vi "subIncrementAndGetProjectItem.vi"(8 "error in (no error)":errorcluster, 11 "BuildManager in":refnum<class "BuildManager.lvclass">) -> (0 "error out":errorcluster, 1 "Valid":bool, 3 "BuildManager out":refnum<class "BuildManager.lvclass">)   [LabVIEW 2019, in "SolutionBuilder.lvlib" / "BuildManager.lvclass"]
uses:
  BuildManager.lvclass
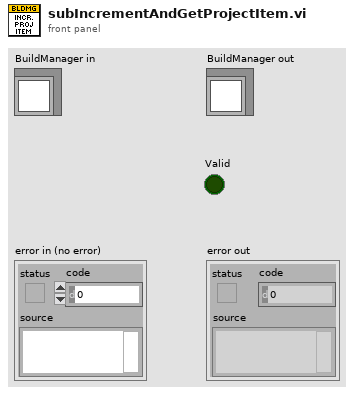
[diagram p1: front panel]
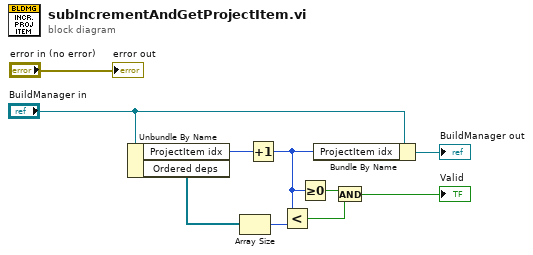
[diagram p0: block diagram]
diagram:
  n1 = Unbundle By Name("BuildManager in") -> ("ProjectItem idx"=w10:i32, "Ordered deps"=w6:refnum<class "ProjectItem.lvclass">[])
  n2 = Array Size(array=w6) -> (size(s)=w5:i32)
  n3 = Increment(x=w10) -> (x+1=w4:i32)
  n4 = Less?(x=w4, y=w5) -> (x < y?=w2:bool)
  n5 = Greater Or Equal To 0?(x=w4) -> (x >= 0?=w3:bool)
  n6 = Bundle By Name(cluster="BuildManager in", "ProjectItem idx"=w4) -> (→"BuildManager out":refnum<class "BuildManager.lvclass">)
  n7 = And(x=w3, y=w2) -> (x .and. y?=→"Valid":bool)
  "error out" <- "error in (no error)"
